vi "SIN_KE622x_.vi"(2 "frequency /HZ":dbl=5.0 min=0.009999999776482582 max=100000.0, 3 "compliance /V":dbl=5.0 min=0.009999999776482582 max=10.0, 4 "entrée d'erreur (pas d'erreur)":errorcluster caption="error in", 5 "amplitude /A":dbl=1.199999957179898e-07 min=-0.10499999672174454 max=0.10499999672174454, 6 "offset /A":dbl min=-0.10000000149011612 max=0.10000000149011612, 7 "VISA GPIB Resource":refnum<visa-resource-name>="GPIB0::4::INSTR") -> (0 "error out":errorcluster, 1 "VISA GPIB Resource out":refnum<visa-resource-name>="GPIB0::4::INSTR")   [LabVIEW 2018]
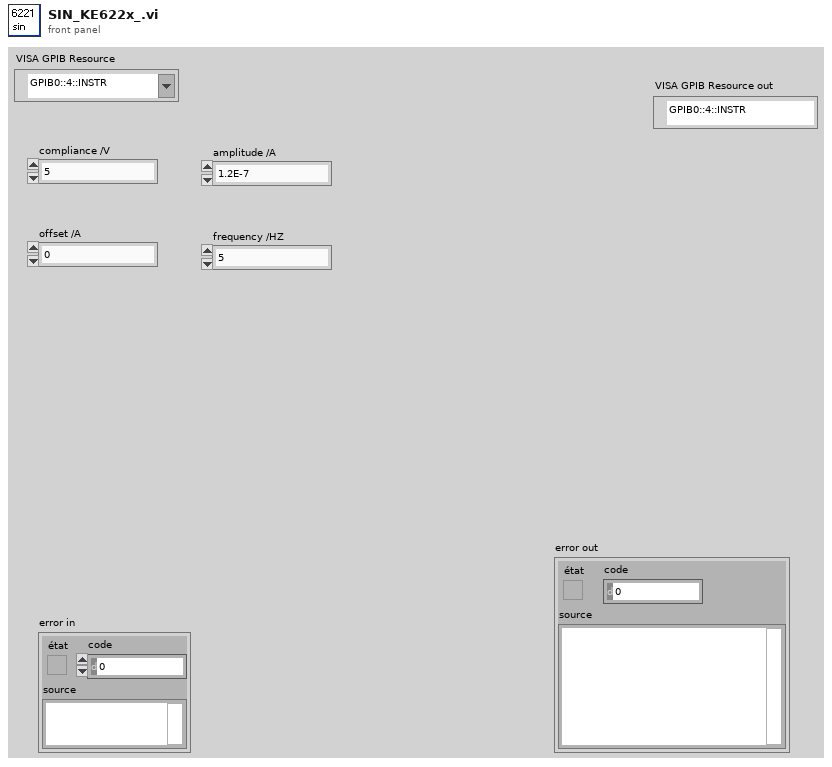
[diagram p1: front panel]
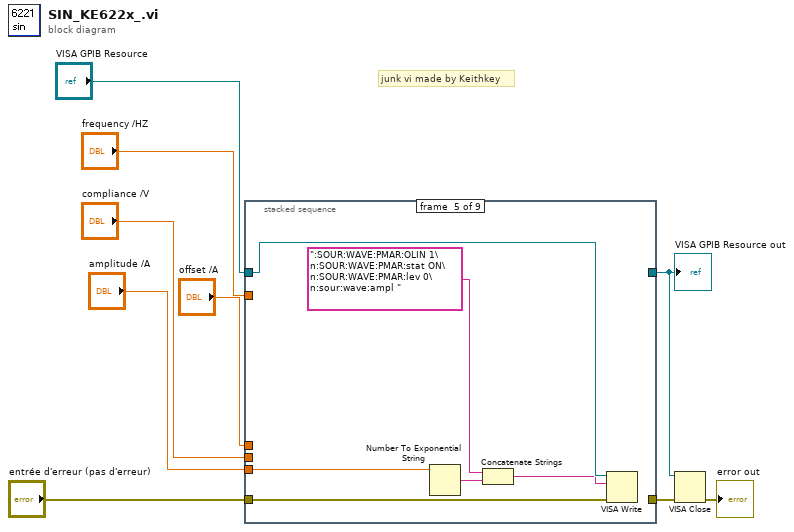
[diagram p0: block diagram]
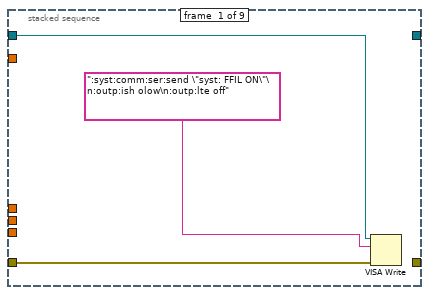
[diagram p2: hidden frame]
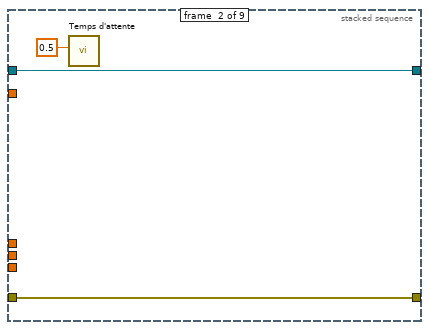
[diagram p3: hidden frame]
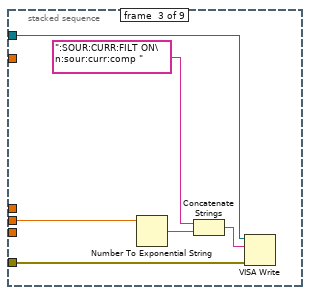
[diagram p4: hidden frame]
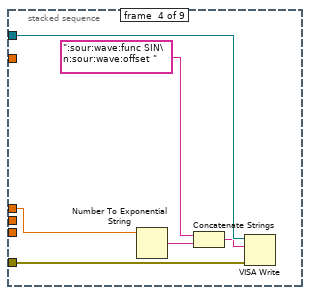
[diagram p5: hidden frame]
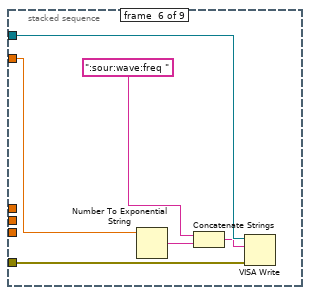
[diagram p6: hidden frame]
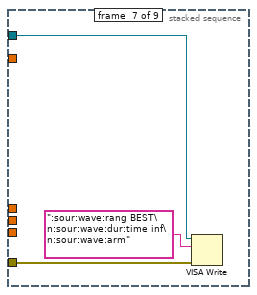
[diagram p7: hidden frame]
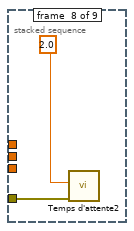
[diagram p8: hidden frame]
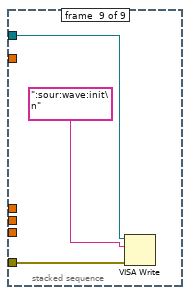
[diagram p9: hidden frame]
diagram:
  # "junk vi made by Keithkey"
  n1 = stacked-sequence {
    tunnel: "VISA GPIB Resource" -> [w11 w14 w21 w27 w33 w39 w42 _ w47]
    tunnel: "entrée d'erreur (pas d'erreur)" -> [w12 w13 w20 w26 w32 w38 w41 w43 w46]
    tunnel: [_ w14 _ _ _ _ _ _ _] -> w1
    tunnel: [_ w13 _ _ _ _ _ _ _] -> w5
    tunnel: "offset /A" -> [_ _ _ w22 _ _ _ _ _]
    tunnel: "compliance /V" -> [_ _ w17 _ _ _ _ _ _]
    tunnel: "amplitude /A" -> [_ _ _ _ w29 _ _ _ _]
    tunnel: "frequency /HZ" -> [_ _ _ _ _ w35 _ _ _]
    frame #0 {
      n2 = VISA Write(VISA resource name=w11, write buffer=":syst:comm:ser:send \"syst: FFIL ON\"\n:outp:ish olow\n:outp:lte off" ("buffer à écrire"), error in (no error)=w12) -> ()  [unwired: 3 out]
    }
    frame #1 {
      n3 = call "Temps d'attente"("Delay Time (s)"=0.5) -> ()  [unwired: 1 in, 10 out]
    }
    frame #2 {
      n4 = Number To Exponential String(number=w17) -> (E-format string=w16:string)  [unwired: 3 out]
      n5 = Concatenate Strings(":SOUR:CURR:FILT ON\n:sour:curr:comp " ("buffer à écrire"), w16) -> (w18:string)
      n6 = VISA Write(VISA resource name=w21, write buffer=w18, error in (no error)=w20) -> ()  [unwired: 3 out]
    }
    frame #3 {
      n7 = Number To Exponential String(number=w22) -> (E-format string=w23:string)  [unwired: 3 out]
      n8 = Concatenate Strings(":sour:wave:func SIN\n:sour:wave:offset " ("buffer à écrire"), w23) -> (w25:string)
      n9 = VISA Write(VISA resource name=w27, write buffer=w25, error in (no error)=w26) -> ()  [unwired: 3 out]
    }
    frame #4 {
      n10 = Number To Exponential String(number=w29) -> (E-format string=w28:string)  [unwired: 3 out]
      n11 = Concatenate Strings(":SOUR:WAVE:PMAR:OLIN 1\n:SOUR:WAVE:PMAR:stat ON\n:SOUR:WAVE:PMAR:lev 0\n:sour:wave:ampl " ("buffer à écrire"), w28) -> (w30:string)
      n12 = VISA Write(VISA resource name=w33, write buffer=w30, error in (no error)=w32) -> ()  [unwired: 3 out]
    }
    frame #5 {
      n13 = Number To Exponential String(number=w35) -> (E-format string=w34:string)  [unwired: 3 out]
      n14 = Concatenate Strings(":sour:wave:freq " ("buffer à écrire"), w34) -> (w36:string)
      n15 = VISA Write(VISA resource name=w39, write buffer=w36, error in (no error)=w38) -> ()  [unwired: 3 out]
    }
    frame #6 {
      n16 = VISA Write(VISA resource name=w42, write buffer=":sour:wave:rang BEST\n:sour:wave:dur:time inf\n:sour:wave:arm" ("buffer à écrire"), error in (no error)=w41) -> ()  [unwired: 3 out]
    }
    frame #7 {
      n17 = call "Temps d'attente2"("error in (no error)"=w43, "Delay Time (s)"=2.0) -> ()  [unwired: 10 out]
    }
    frame #8 {
      n18 = VISA Write(VISA resource name=w47, write buffer=":sour:wave:init\n" ("buffer à écrire"), error in (no error)=w46) -> ()  [unwired: 3 out]
    }
  }
  "VISA GPIB Resource out" <- w1
  n19 = VISA Close(VISA resource name=w1, error in (no error)=w5) -> (error out=→"error out":errorcluster)
